vi "find last occupied cell.vi"(0 "data":string[][](array[string]), 1 "Active Sheet":string, 5 "Header Rows to remove":i32=2, 7 "sub array start":cluster{"row":i32, "column":i32}, 11 "error in (no error)":errorcluster) -> (4 "row max value":i32, 6 "column max value":i32, 8 "last occupied cell":cluster{"row":i32, "column":i32}, 10 "last occupied cell's name":string, 13 "start of last occupied row":cluster{"row":i32, "column":i32}, 14 "start of last occupied row":string, 15 "error out":errorcluster)   [LabVIEW 2016]
uses:
  <vilib>/addons/_office/NI_ReportGenerationToolkit.lvlib
panel:
  out "size(s) 2":i32[](array[numeric])
  out "Array":i32[][](array[numeric])
  out "subarray 2":string[][](array[string])
  out "size(s)":i32[](array[numeric])
  out "Initial size(s)":i32[](array[numeric])
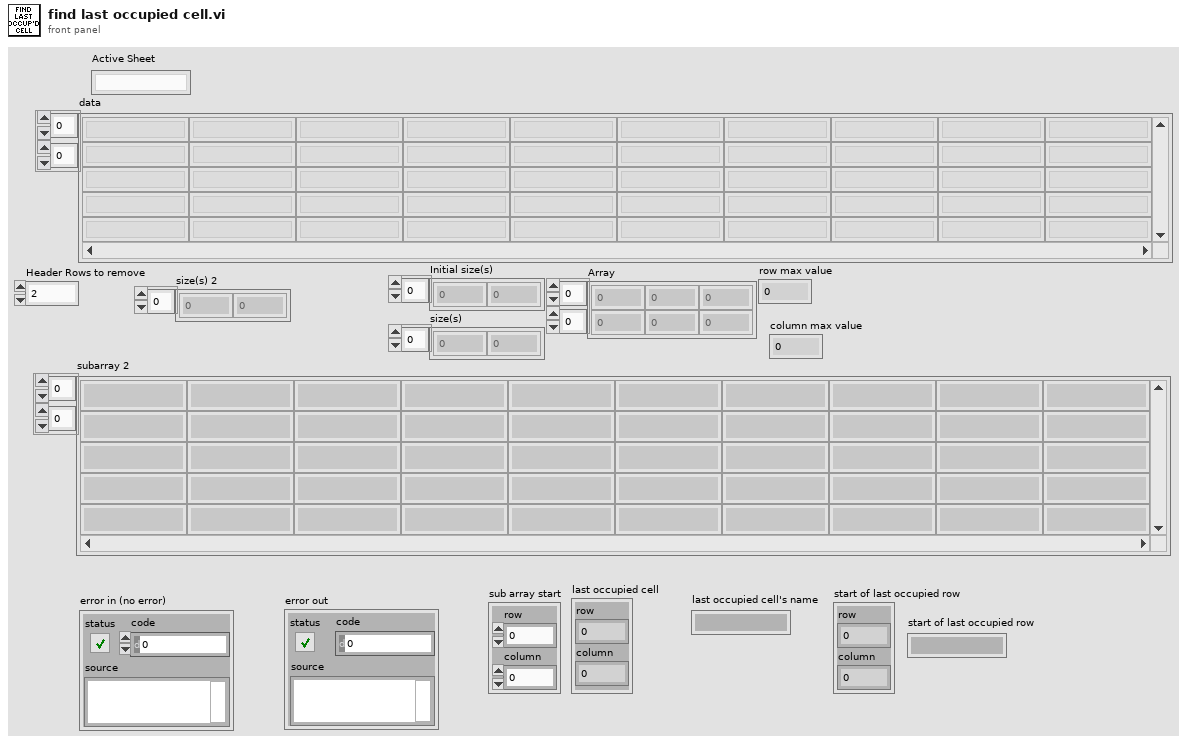
[diagram p1: front panel]
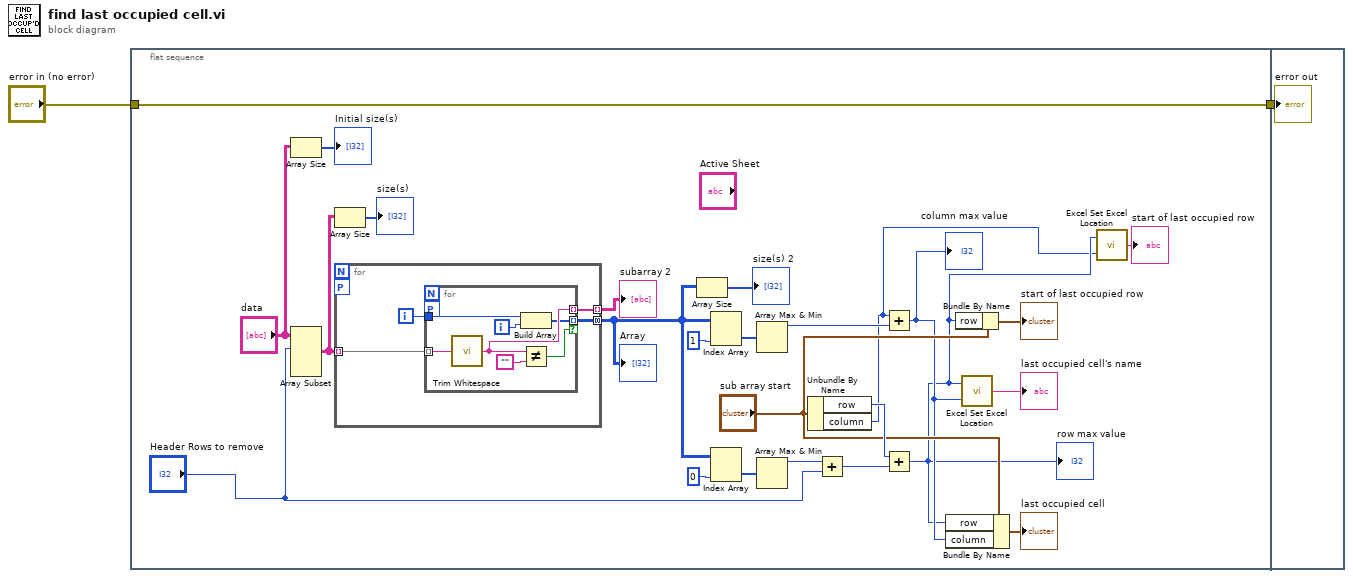
[diagram p0: block diagram]
diagram:
  n1 = flat-sequence {
    tunnel: "error in (no error)" -> [w16]
    tunnel: [w16] -> w1
    tunnel: w1 -> [w39]
    frame #0 {
      n2 = Array Size(array="data") -> (size(s)=→"Initial size(s)":i32[])
      n3 = Array Subset(array="data", index (row)="Header Rows to remove") -> (w24:string[][])  [unwired: 3 in]
      n4 = Array Size(array=w24) -> (size(s)=→"size(s)":i32[])
      n5 = for {
        tunnel: w24 -> [w31] mode=indexing
        tunnel: [w30] -> w23 mode=indexing
        tunnel: [w28] -> w21 mode=concatenating
        workers-P: _ -> [_]
        i -> [w29]
        n6 = for {
          tunnel: w31 -> [w38] mode=indexing
          tunnel: [w36] -> w30 mode=indexing
          tunnel: [w33] -> w28 mode=indexing if=w32
          tunnel: w29 -> [w35]
          workers-P: _ -> [_]
          i -> [w34]
          n7 = call <vilib>:"Trim Whitespace.vi"("string"=w38) -> ("trimmed string"=w36:string)  [unwired: 1 in]
          n8 = Build Array(w35, w34) -> (w33:i32[])
          n9 = Not Equal?(x=w36, y="") -> (x != y?=w32:bool)
        }
      }
      "subarray 2" <- w23
      "Array" <- w21
      n10 = Array Size(array=w21) -> (size(s)=→"size(s) 2":i32[])
      n11 = Index Array(array=w21, index (col)=1 ("index")) -> (element=w17:i32[])  [unwired: 1 in]
      n12 = Index Array(array=w21, index (col)=0 ("index")) -> (element=w18:i32[])  [unwired: 1 in]
      n13 = Array Max & Min(array=w17) -> (max value=w11:i32)  [unwired: 3 out]
      n14 = Array Max & Min(array=w18) -> (max value=w15:i32)  [unwired: 3 out]
      n15 = Unbundle By Name("sub array start") -> ("row"=w12:i32, "column"=w5:i32)
      n16 = Add(x=w15, y="Header Rows to remove") -> (x+y=w13:i32)
      n17 = Add(x=w5, y=w11) -> (x+y=w7:i32)
      "column max value" <- w7
      n18 = Add(x=w12, y=w13) -> (x+y=w6:i32)
      "row max value" <- w6
      n19 = Bundle By Name(cluster="sub array start", "row"=w6, "column"=w7) -> (→"last occupied cell":cluster{"row":i32, "column":i32})
      n20 = Bundle By Name(cluster="sub array start", "row"=w6) -> (→"start of last occupied row":cluster{"row":i32, "column":i32})
      n21 = call <vilib>:"Excel Set Excel Location.vi"("column"=w7, "row"=w6) -> ("cell's name"=→"last occupied cell's name":string)
      n22 = call <vilib>:"Excel Set Excel Location.vi"("column"=w5, "row"=w6) -> ("cell's name"=→"start of last occupied row":string)
    }
    frame #1 {
      "error out" <- w39
    }
  }
